vi "gyro_binary_get_data.vi"(8 "error in":errorcluster, 10 "all in one package in":T1 {"time informations"."length" format="%<%H:%M:%S%3u>t"; "actigraph settings"."id" format="%02d"; "actigraph settings"."xlRange" format="%02x"; "actigraph settings"."ODR" format="%02x"}, 11 "pages excluding first and last page":u8[](array[numeric])) -> (0 "error out":errorcluster, 3 "all in one package out":T1 {"time informations"."length" format="%<%H:%M:%S%3u>t"; "actigraph settings"."id" format="%02d"; "actigraph settings"."xlRange" format="%02x"; "actigraph settings"."ODR" format="%02x"})   [LabVIEW 2019]
uses:
  Controls/gyro_control_measurement_settings.ctl
  Controls/gyro_control_memory_structure.ctl
  Controls/gyro_control_time_informations.ctl
  Controls/gyro_control_measurement_data.ctl
  Controls/gyro_control_all_in_one_package.ctl
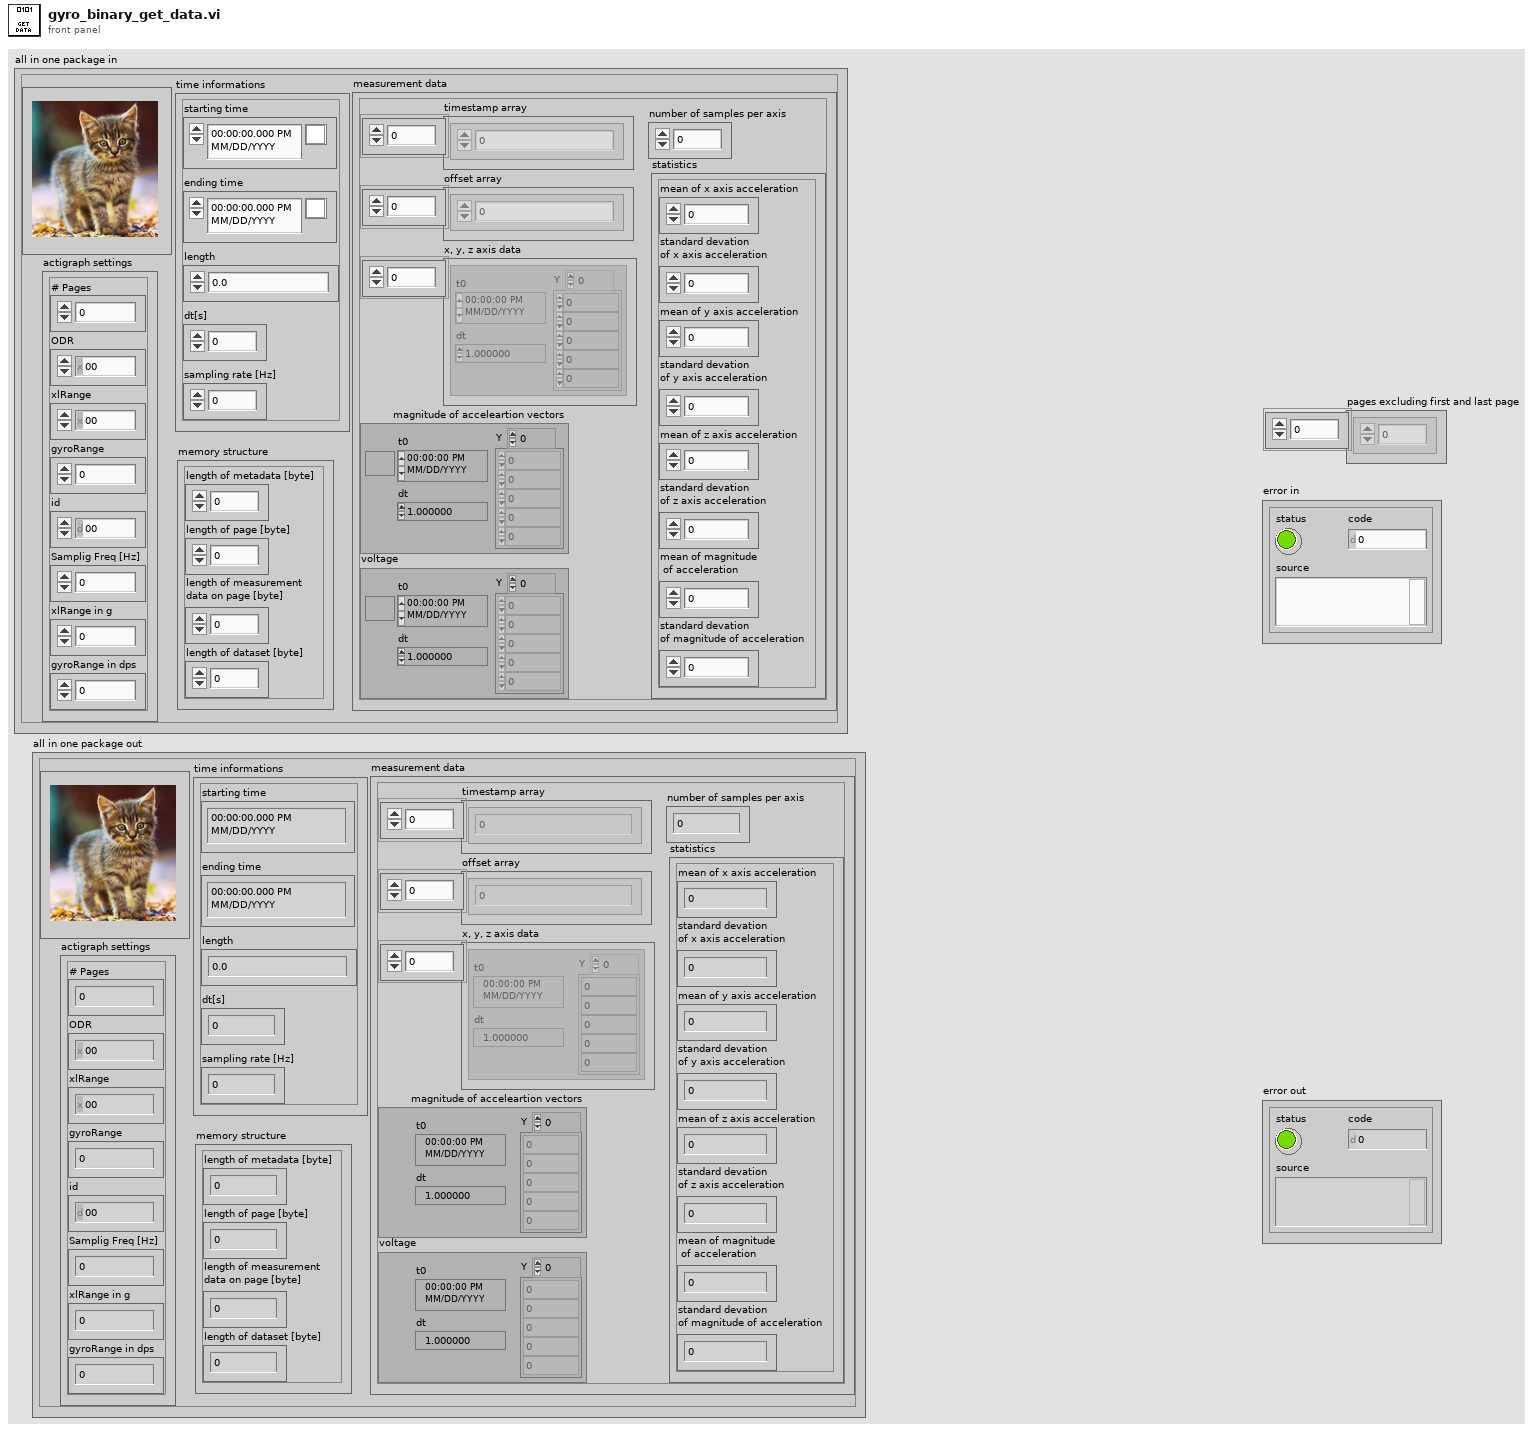
[diagram p1: front panel]
types:
  T1 = typedef "gyro_control_all_in_one_package.ctl" = cluster{"measurement data":T2, "actigraph settings":T3, "memory structure":T4, "time informations":T5}
  T2 = typedef "gyro_control_measurement_data.ctl" = cluster{"number of samples per axis":i32, "timestamp array":dbl[], "offset array":dbl[], "x, y, z axis data":waveform(dbl)[], "magnitude of acceleartion vectors":waveform(dbl), "statistics":cluster{"mean of x axis acceleration":dbl, "standard devation \nof x axis acceleration":dbl, "mean of y axis acceleration":dbl, "standard devation \nof y axis acceleration":dbl, "mean of z axis acceleration":dbl, "standard devation \nof z axis acceleration":dbl, "mean of magnitude\n of acceleration":dbl, "standard devation \nof magnitude of acceleration":dbl}, "voltage":waveform(dbl)}
  T3 = typedef "gyro_control_measurement_settings.ctl" = cluster{"# Pages":i32, "ODR":u8, "xlRange":u8, "gyroRange":u8, "id":u8, "Samplig Freq [Hz]":dbl, "xlRange in g":dbl, "gyroRange in dps":dbl}
  T4 = typedef "gyro_control_memory_structure.ctl" = cluster{"length of metadata [byte]":i32, "length of page [byte]":i32, "length of measurement \ndata on page [byte]":i32, "length of dataset [byte]":i32}
  T5 = typedef "gyro_control_time_informations.ctl" = cluster{"starting time":timestamp, "ending time":timestamp, "dt[s]":dbl, "sampling rate [Hz]":dbl, "length":dbl}
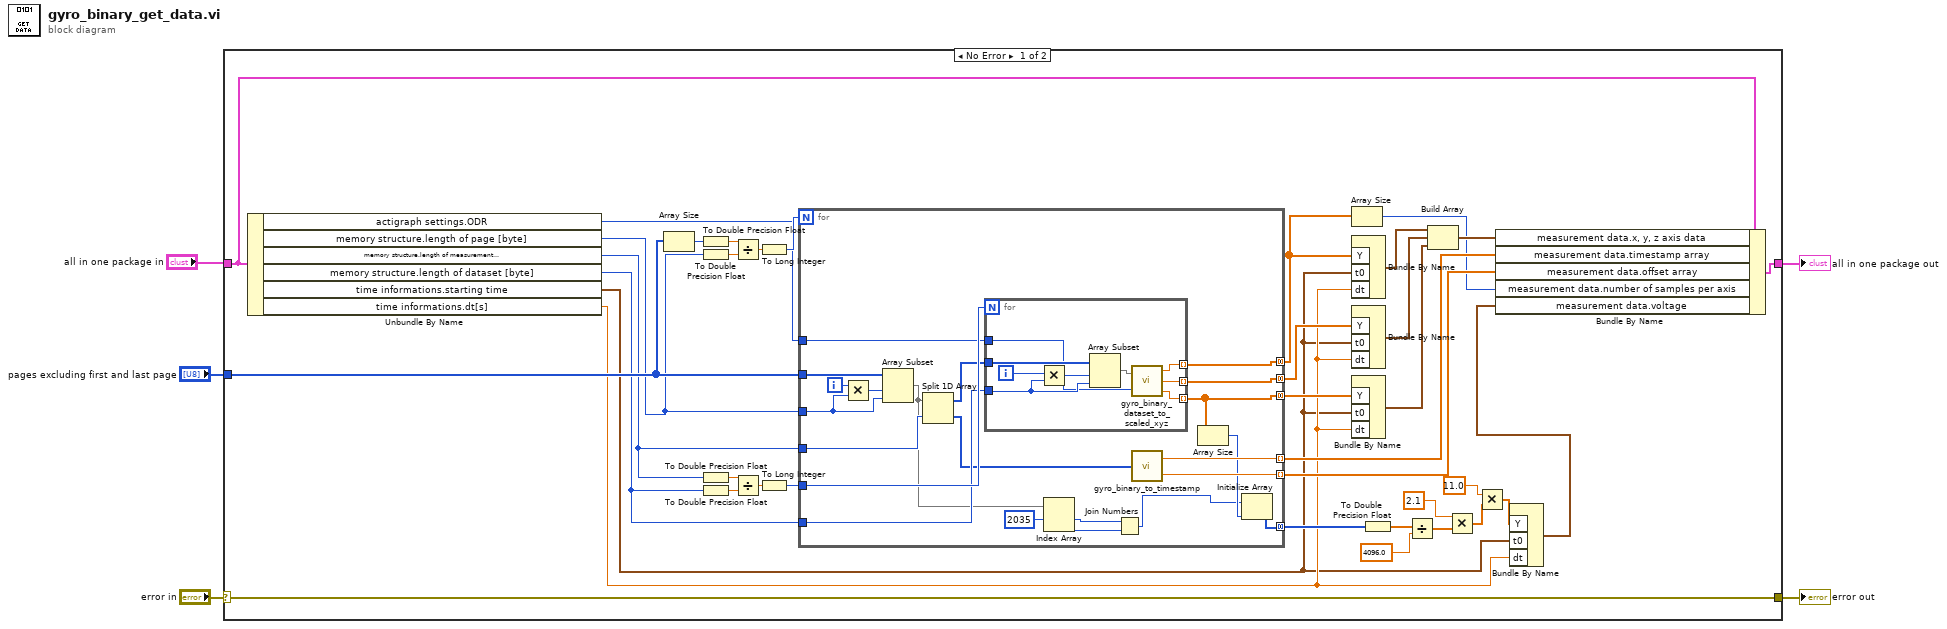
[diagram p0: block diagram]
diagram:
  n1 = case shown="No Error" "error in" {
    selector: "error in" -> [w43 w76]
    tunnel: "pages excluding first and last page" -> [w38 _]
    tunnel: [w43 w76] -> w4
    tunnel: "all in one package in" -> [w24 w75]
    tunnel: [w22 w75] -> w1
    frame No Error {
      n2 = Unbundle By Name(w24) -> ("actigraph settings.ODR"=w32:u8, "memory structure.length of page [byte]"=w31:i32, "memory structure.length of measurement \ndata on page [byte]"=w30:i32, "memory structure.length of dataset [byte]"=w18:i32, "time informations.starting time"=w10:timestamp, "time informations.dt[s]"=w11:dbl)
      n3 = Array Size(array=w38) -> (size(s)=w42:i32)
      n4 = To Double Precision Float(number=w42) -> (double precision float=w39:dbl)
      n5 = To Double Precision Float(number=w31) -> (double precision float=w40:dbl)
      n6 = To Double Precision Float(number=w30) -> (double precision float=w34:dbl)
      n7 = To Double Precision Float(number=w18) -> (double precision float=w35:dbl)
      n8 = Divide(x=w39, y=w40) -> (x/y=w41:dbl)
      n9 = Divide(x=w34, y=w35) -> (x/y=w36:dbl)
      n10 = To Long Integer(number=w41) -> (32bit integer=w37:i32)
      n11 = To Long Integer(number=w36) -> (32bit integer=w33:i32)
      n12 = for {
        N: w37 -> [_]
        tunnel: [w65] -> w29 mode=concatenating
        tunnel: [w64] -> w28 mode=concatenating
        tunnel: [w47] -> w17 mode=concatenating
        tunnel: w30 -> [w60]
        tunnel: w38 -> [w62]
        tunnel: w31 -> [w57]
        tunnel: w33 -> [w61]
        tunnel: w18 -> [w56]
        tunnel: w32 -> [w55]
        tunnel: [w53] -> w21 mode=indexing
        tunnel: [w52] -> w20 mode=indexing
        tunnel: [w44] -> w16 mode=concatenating
        i -> [w58]
        # "Iterate through pages (excluding first page). One page is 2048 bytes long and the first 2028 bytes holds the measurement data of x, y, z axis.  Each and every measurement value is stored on 2 bytes, therefore 6 bytes contains the x, y, z dataset of an exact moment. Since one page contains 2028 bytes and a dataset of one moment is 6 bytes, one page holds a total of 338 datasets. The measurement values are automatically scaled by the measurement interval (e.g. +-8g). The first 6 bytes of the remaining 20 bytes on page contains the timestamp. Timestamps indicate the moment of last dataset stored on page.  Every iteration makes an array of x, y, z (separately) measurement values, in the end they will be concatenated and ready to further modifications."
        n13 = Multiply(x=w58, y=w57) -> (x*y=w63:i32)
        n14 = Array Subset(array=w62, index=w63, length=w57) -> (w51:u8[])
        n15 = Split 1D Array(array=w51, index=w60) -> (first subarray=w59:u8[], second subarray=w54:u8[])
        n16 = for {
          N: w61 -> [_]
          tunnel: w59 -> [w74]
          tunnel: [w71] -> w65 mode=indexing
          tunnel: [w72] -> w64 mode=indexing
          tunnel: [w70] -> w47 mode=indexing
          tunnel: w56 -> [w67]
          tunnel: w55 -> [w66]
          i -> [w68]
          # "Iterate through datasets on page."
          n17 = Multiply(x=w68, y=w67) -> (x*y=w73:i32)
          n18 = Array Subset(array=w74, index=w73, length=w67) -> (w69:u8[])
          n19 = call "gyro_binary_dataset_to_scaled_xyz.vi"("binarySet"=w69, 1:w66) -> ("x axis value"=w71:dbl, "y axis value"=w72:dbl, "z axis value"=w70:dbl)
        }
        n20 = Index Array(array=w51, index #1=2035 ("index")) -> (element #1=w49:u8, element #2=w48:u8)  [unwired: 1 in]
        n21 = Join Numbers(hi=w49, lo=w48) -> ((hi.lo)=w45:u16)
        n22 = call "gyro_binary_to_timestamp.vi"("binaryTimestampWithOffset"=w54) -> ("timestamp"=w53:dbl, "offset"=w52:dbl)
        n23 = Array Size(array=w47) -> (size(s)=w46:i32)
        n24 = Initialize Array(w45, w46) -> (w44:u16[])
      }
      n25 = Array Size(array=w29) -> (size(s)=w19:i32)
      n26 = Bundle By Name("Y"=w29, "t0"=w10, "dt"=w11) -> (w27:waveform(dbl))  [unwired: 1 in]
      n27 = Bundle By Name("Y"=w28, "t0"=w10, "dt"=w11) -> (w26:waveform(dbl))  [unwired: 1 in]
      n28 = Bundle By Name("Y"=w17, "t0"=w10, "dt"=w11) -> (w25:waveform(dbl))  [unwired: 1 in]
      n29 = To Double Precision Float(number=w16) -> (double precision float=w15:dbl[])
      n30 = Divide(x=w15, y=4096.0 ("time informations.dt[s]")) -> (x/y=w13:dbl[])
      n31 = Build Array(w27, w26, w25) -> (w23:waveform(dbl)[])
      n32 = Multiply(x=2.1 ("time informations.dt[s]"), y=w13) -> (x*y=w7:dbl[])
      n33 = Multiply(x=11.0 ("time informations.dt[s]"), y=w7) -> (x*y=w6:dbl[])
      n34 = Bundle By Name("Y"=w6, "t0"=w10, "dt"=w11) -> (w9:waveform(dbl))  [unwired: 1 in]
      n35 = Bundle By Name(cluster=w24, "measurement data.x, y, z axis data"=w23, "measurement data.timestamp array"=w21, "measurement data.offset array"=w20, "measurement data.number of samples per axis"=w19, "measurement data.voltage"=w9) -> (w22:T1)
    }
    frame Error {
    }
  }
  "error out" <- w4
  "all in one package out" <- w1
